vi "Function Selected.vi"(7 "Module Name":string, 8 "error in":errorcluster, 9 "Item Name":string, 10 "ItemIndex":i32, 11 "Module ID":i32=-1) -> (0 "error out":errorcluster)   [LabVIEW 2018, in "ModuleInterface.lvlib"]
doc: "广播双击选中的功能项的索引\n_____\nCreated using DQMH Event Scripter 7.0.1.1316."
uses:
  ModuleInterface.lvlib
  FunctionSelected Argument--cluster.ctl
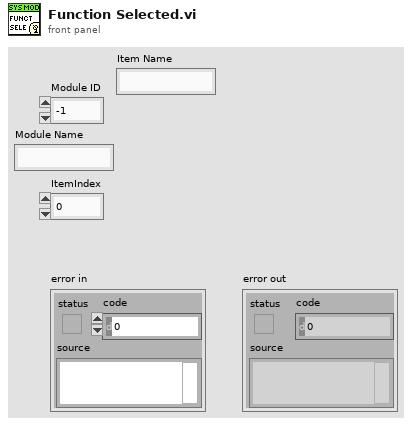
[diagram p1: front panel]
types:
  T1 = typedef "ModuleInterface.lvlib/FunctionSelected Argument--cluster.ctl" = cluster{"Module ID":i32, "Module Name":string, "SelectedItem":i32, "Item Name":string}
  T2 = typedef "ModuleInterface.lvlib/Broadcast Events--cluster.ctl" = cluster{"Module Did Init":refnum<user-event>, "Status Updated":refnum<user-event>, "Error Reported":refnum<user-event>, "Module Did Stop":refnum<user-event>, "Update Module Execution Status":refnum<user-event>, "Function Selected":refnum<user-event>, "Window Size Changed":refnum<user-event>}
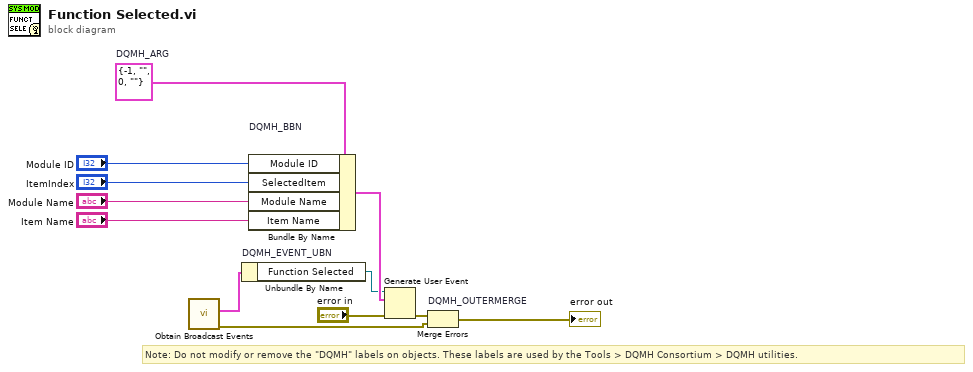
[diagram p0: block diagram]
diagram:
  w7 = T1 {"Module ID"=-1, "Module Name"="", "SelectedItem"=0, "Item Name"=""}  # DQMH_ARG
  # "Note: Do not modify or remove the \"DQMH\" labels on objects. These labels are used by the Tools > DQMH Consortium > DQMH utilities."
  n1 = call "Obtain Broadcast Events.vi"() -> ("error out"=w4:errorcluster, "ModuleInterface Broadcast Events"=w3:T2)  [unwired: 10 in]
  n2 = Unbundle By Name "DQMH_EVENT_UBN"(w3) -> ("Function Selected"=w9:refnum<user-event>)
  n3 = Bundle By Name "DQMH_BBN"(cluster=w7, "Module ID"="Module ID", "SelectedItem"="ItemIndex", "Module Name"="Module Name", "Item Name"="Item Name") -> (w10:T1)
  n4 = Generate User Event(user event=w9, event data cluster=w10, error in="error in") -> (error out=w8:errorcluster)  [unwired: 1 in, 1 out]
  n5 = Merge Errors "DQMH_OUTERMERGE"(w8, w4) -> (→"error out":errorcluster)
